vi "TEST FGV User Event Reference Manager.vi"(8 "error in (no error)":errorcluster) -> (0 "error out":errorcluster)   [LabVIEW 2009]
doc: "This is one of two stub VIs that will be completed in the exercise so that you can test the operation of the FGV User Event Reference Manager.\n\nAAL 9/09"
uses:
  Shared/QDMH Poly VIs/QDMH POLY Enqueue String.vi
panel:
  in  "Queue Name":string
  in  "Fire User Event":bool
  in  "User Event Ref to Act Upon":u16(ring)
  in  "Delete User Event":bool
  in  "Add User Event":bool
  out "Message Display":string
  in  "Cancel":bool
  in  "OK":bool
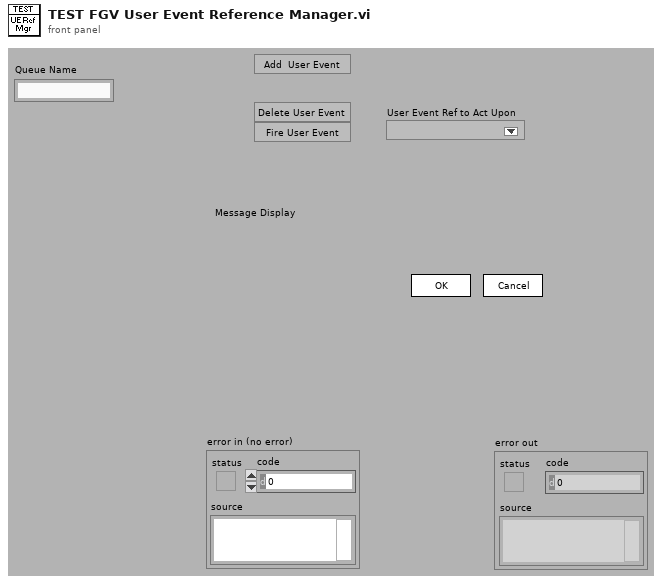
[diagram p1: front panel]
types:
  T1 = cluster{"Operator Name":string, "Current VI's Path":path, "# User Event  Refs":i32, "User Event #":i32, "User Event Names":string[], "User Event to Act Upon":i32}
  T2 = cluster{"User Event Name":string, "Variant":variant}
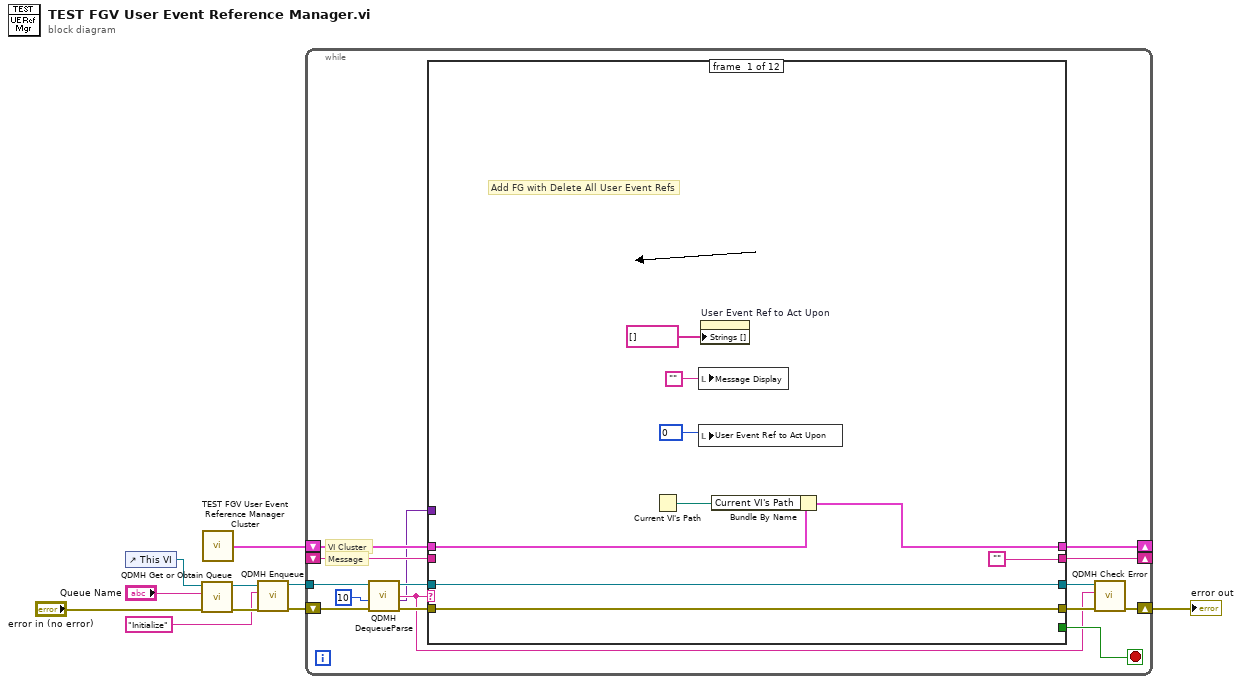
[diagram p0: block diagram]
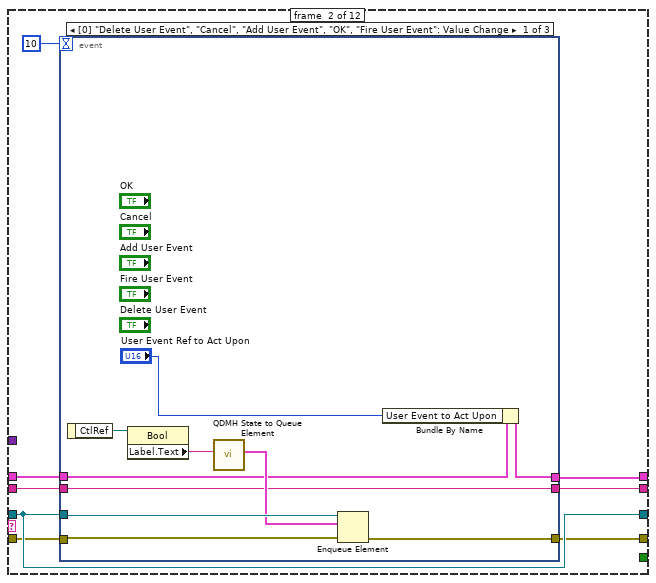
[diagram p2: hidden frame]
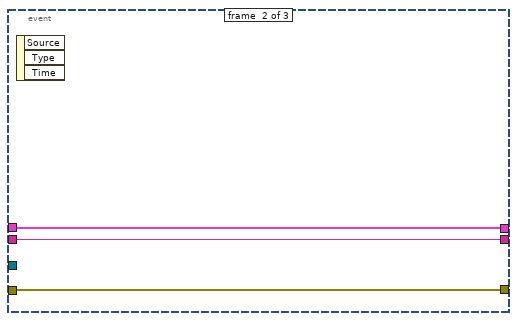
[diagram p3: hidden frame]
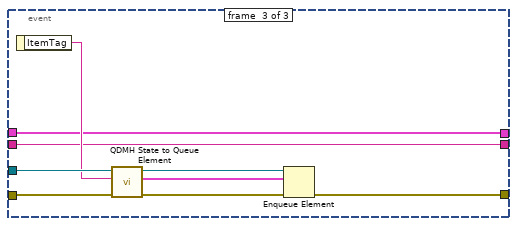
[diagram p4: hidden frame]
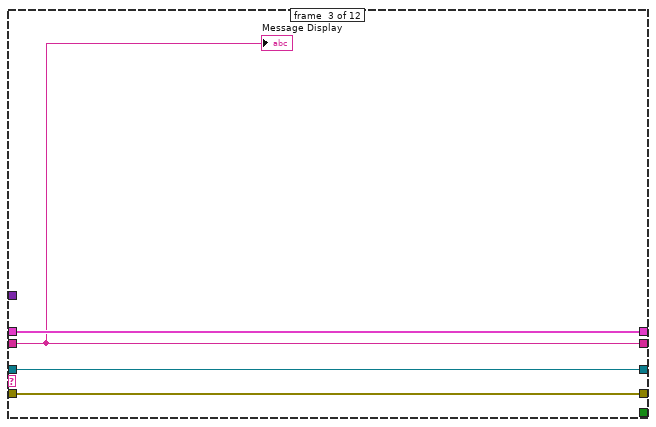
[diagram p5: hidden frame]
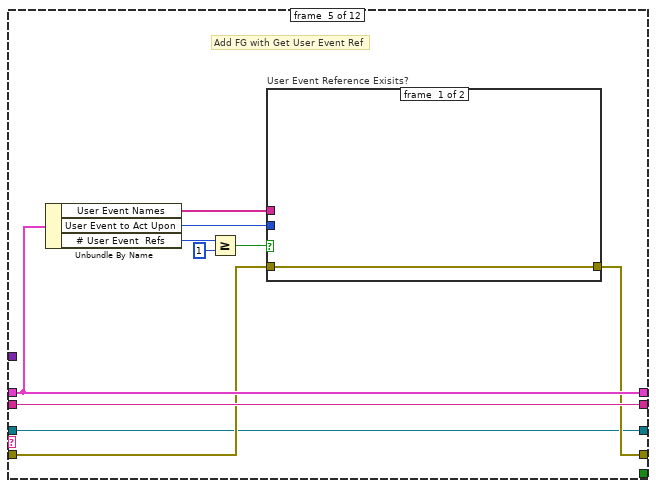
[diagram p7: hidden frame]
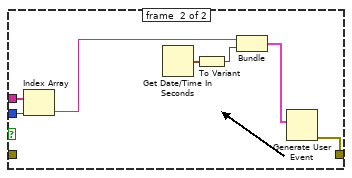
[diagram p8: hidden frame]
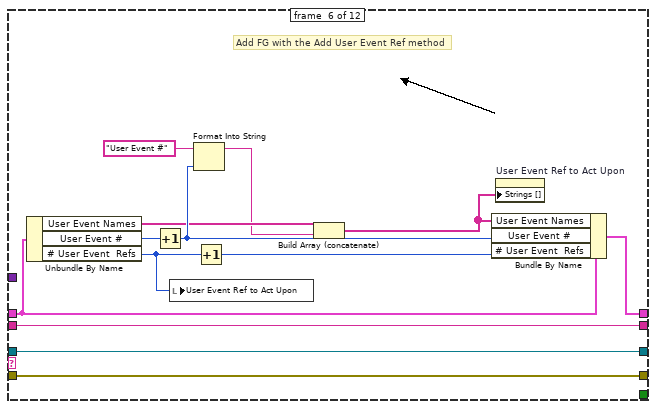
[diagram p9: hidden frame]
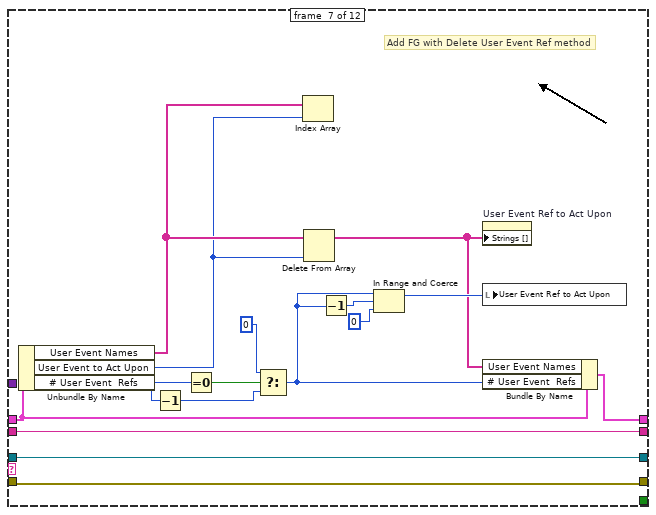
[diagram p10: hidden frame]
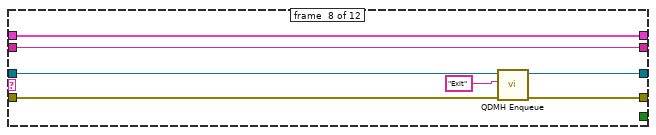
[diagram p11: hidden frame]
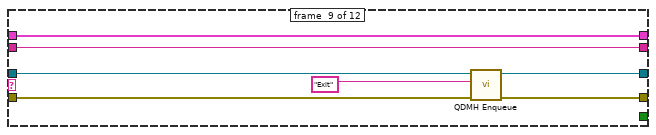
[diagram p12: hidden frame]
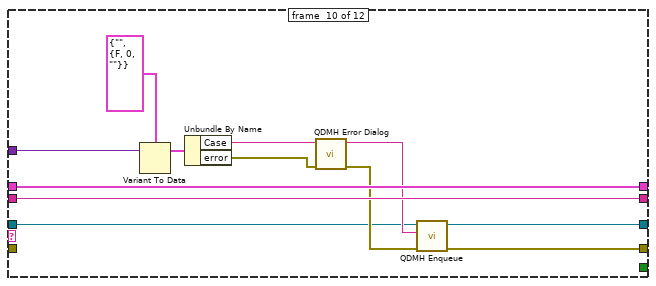
[diagram p13: hidden frame]
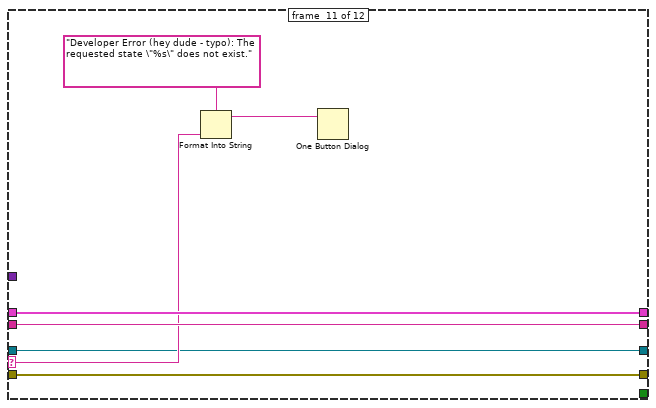
[diagram p14: hidden frame]
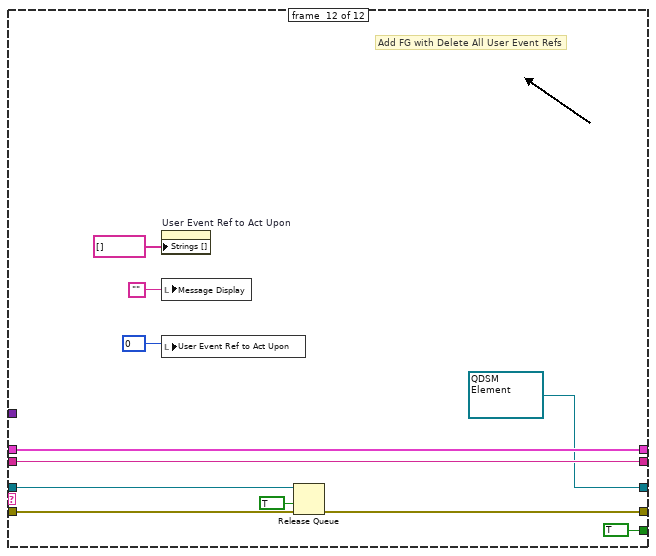
[diagram p15: hidden frame]
diagram:
  n1 = control-ref of="This VI"() -> (w2:refnum<vi>)
  n2 = call "QDMH Get or Obtain Queue.vi"("error in (no error)"="error in (no error)", "Queue Name"="Queue Name", "VI Refnum"=w2) -> ("error out"=w6:errorcluster, "queue out"=w9:refnum<queue>)  [unwired: 7 out]
  n3 = call "TEST FGV User Event Reference Manager Cluster.vi"() -> ("Cluster"=w8:T1)
  n4 = call-poly "QDMH Enqueue.vi"("error in (no error)"=w6, "State"="Initialize" ("element"), "queue"=w9) -> ("error out"=w7:errorcluster, "queue out"=w10:refnum<queue>)  [unwired: 7 out]
  n5 = while {
    tunnel: w10 -> [w21]
    shift-left: w8 -> [w22]
    shift-right: [w23] -> _
    shift-left: _ -> [w24]
    shift-right: [w15] -> _
    shift-right: [w13] -> w4
    shift-left: w7 -> [w17]
    stop <- w25 stop-if-true
    # "VI Cluster"
    # "Message"
    n6 = call "QDMH DequeueParse.vi"("error in (no error)"=w17, "Timeout"=10 ("ms timeout (-1)"), "queue"=w21) -> ("error out"=w18:errorcluster, "Variant Data"=w11:variant, "State"=w12:string, "queue out"=w19:refnum<queue>)  [unwired: 5 out]
    n7 = case shown="\"Initialize\"" w12 {
      selector: w12 -> [_ _ _ _ _ _ _ _ _ _ w147 _]
      tunnel: w19 -> [w26 w42 w63 w67 w71 w90 w102 w124 w131 w133 w144 w152]
      tunnel: [_ _ _ _ _ _ _ _ _ _ _ TRUE] -> w25
      tunnel: ["" w36 w65 w70 w80 w101 w117 w123 w130 w143 w150 w160] -> w15
      tunnel: w24 -> [_ w37 w65 w70 w80 w101 w117 w123 w130 w143 w150 w160]
      tunnel: [w32 w35 w66 w69 w79 w98 w115 w122 w129 w142 w149 w159] -> w23
      tunnel: w22 -> [w33 w38 w66 w69 w79 w99 w116 w122 w129 w142 w149 w159]
      tunnel: w18 -> [w34 w41 w64 w68 w76 w91 w104 w121 w128 _ w146 w157]
      tunnel: [w34 w40 w64 w68 w75 w91 w104 w120 w127 w134 w146 w156] -> w16
      tunnel: [w26 w42 w63 w67 w71 w90 w102 w118 w125 w135 w144 refnum<queue> refnum ("queue out")] -> w14
      tunnel: w11 -> [_ _ _ _ _ _ _ _ _ w132 _ _]
      frame #0 {
        w27 = u16 0 items=[""] ("Queue to Delete")
        # "Add FG with Delete All User Event Refs"
        n8 = Current VI's Path() -> (path=w31:path)
        n9 = local write "Message Display"("") -> ()
        n10 = local write "User Event Ref to Act Upon"(w27) -> ()
        n11 = property on="User Event Ref to Act Upon" class="Ring (strict)"("Strings []"=string[] []) -> ()  [unwired: 2 in, 2 out]
        n12 = Bundle By Name(cluster=w33, "Current VI's Path"=w31) -> (w32:T1)
      }
      frame #1 {
        n13 = event shown="[0] \"Delete User Event\", \"Cancel\", \"Add User Event\", \"OK\", \"Fire User Event\": Value Change" {
          selector: _ -> [_ _ _]
          dyn-events: _ -> [_ _ _]
          timeout: 10 -> [_ _ _]
          tunnel: w42 -> [w51 _ w62]
          tunnel: [w50 w55 w60] -> w40
          tunnel: w41 -> [w49 w55 w61]
          tunnel: w38 -> [w45 w54 w57]
          tunnel: w37 -> [w46 w53 w56]
          tunnel: [w44 w54 w57] -> w35
          tunnel: [w46 w53 w56] -> w36
          event #0 {
            n14 = event-data() -> ("CtlRef"=w52:refnum<vi>)  [unwired: 1 out]
            n15 = property class="Bool"(reference=w52) -> ("Label.Text"=w48:string)  [unwired: 1 in, 2 out]
            n16 = call "QDMH State to Queue Element.vi"("State"=w48) -> ("QDSM Element"=w47:cluster{"State":string, "Variant Data":variant})  [unwired: 10 out]
            n17 = Enqueue Element(queue=w51, element=w47, error in (no error)=w49) -> (error out=w50:errorcluster)  [unwired: 3 out]
            n18 = Bundle By Name(cluster=w45, "User Event to Act Upon"="User Event Ref to Act Upon") -> (w44:T1)
          }
          event #1 {
            n19 = event-data() -> ()  [unwired: 4 out]
          }
          event #2 {
            n20 = event-data() -> ("ItemTag"=w59:string)  [unwired: 1 out]
            n21 = call "QDMH State to Queue Element.vi"("State"=w59) -> ("QDSM Element"=w58:cluster{"State":string, "Variant Data":variant})  [unwired: 10 out]
            n22 = Enqueue Element(queue=w62, element=w58, error in (no error)=w61) -> (error out=w60:errorcluster)  [unwired: 3 out]
          }
        }
      }
      frame #2 {
        "Message Display" <- w65
      }
      frame #3 {
      }
      frame #4 {
        # "Add FG with Get User Event Ref"
        n23 = Unbundle By Name(w79) -> ("User Event Names"=w78:string[], "User Event to Act Upon"=w77:i32, "# User Event  Refs"=w74:i32)
        n24 = Greater Or Equal?(x=w74, y=1) -> (x >= y?=w72:bool)
        n25 = case "User Event Reference Exisits?" shown="True" w72 {
          tunnel: w78 -> [_ w88]
          tunnel: w77 -> [_ w84]
          tunnel: w76 -> [w81 _]
          tunnel: [w81 w83] -> w75
          frame #0 {
          }
          frame #1 {
            n26 = Index Array(array=w88, index=w84) -> (element=w82:string)
            n27 = Get Date/Time In Seconds() -> (seconds since 1Jan1904=w87:timestamp)
            n28 = To Variant(anything=w87) -> (Variant=w86:variant)
            n29 = Bundle("User Event Name"=w82, "Variant"=w86) -> (w85:T2)  [unwired: 1 out]
            n30 = Generate User Event(event data cluster=w85) -> (error out=w83:errorcluster)  [unwired: 2 in, 1 out]
          }
        }
      }
      frame #5 {
        # "Add FG with the Add User Event Ref method"
        n31 = Unbundle By Name(w99) -> ("User Event Names"=w94:string[], "User Event #"=w97:i32, "# User Event  Refs"=w92:i32)
        n32 = Increment(x=w97) -> (x+1=w96:i32)
        n33 = local write "User Event Ref to Act Upon"(w92) -> ()
        n34 = Format Into String(initial string="User Event #", w96) -> (resulting string=w89:string)  [unwired: 2 in, 1 out]
        n35 = Increment(x=w92) -> (x+1=w95:i32)
        n36 = Build Array (concatenate)(w94, w89) -> (w93:string[])
        n37 = Bundle By Name(cluster=w99, "User Event Names"=w93, "User Event #"=w96, "# User Event  Refs"=w95) -> (w98:T1)
        n38 = property on="User Event Ref to Act Upon" class="Ring (strict)"("Strings []"=w93) -> ()  [unwired: 2 in, 2 out]
      }
      frame #6 {
        # "Add FG with Delete User Event Ref method"
        n39 = Unbundle By Name(w116) -> ("User Event Names"=w106:string[], "User Event to Act Upon"=w105:i32, "# User Event  Refs"=w113:i32)
        n40 = Decrement(x=w113) -> (x-1=w111:i32)
        n41 = Equal To 0?(x=w113) -> (x = 0?=w114:bool)
        n42 = Select(t=0 ("# Queue Refs"), s=w114, f=w111) -> (s? t:f=w108:i32)
        n43 = Index Array(array=w106, index=w105) -> ()  [unwired: 1 out]
        n44 = Delete From Array(array=w106, index=w105) -> (array with subset deleted=w103:string[])  [unwired: 1 in, 1 out]
        n45 = Decrement(x=w108) -> (x-1=w110:i32)
        n46 = In Range and Coerce(upper limit=w108, x=w110, lower limit=0) -> (coerced(x)=w107:i32)  [unwired: 1 out]
        n47 = property on="User Event Ref to Act Upon" class="Ring (strict)"("Strings []"=w103) -> ()  [unwired: 2 in, 2 out]
        n48 = local write "User Event Ref to Act Upon"(w107) -> ()
        n49 = Bundle By Name(cluster=w116, "User Event Names"=w103, "# User Event  Refs"=w108) -> (w115:T1)
      }
      frame #7 {
        n50 = call-poly "QDMH Enqueue.vi"("error in (no error)"=w121, "State"="Exit" ("New State"), "queue"=w124) -> ("error out"=w120:errorcluster, "queue out"=w118:refnum<queue>)  [unwired: 7 out]
      }
      frame #8 {
        n51 = call-poly "QDMH Enqueue.vi"("error in (no error)"=w128, "State"="Exit" ("New State"), "queue"=w131) -> ("error out"=w127:errorcluster, "queue out"=w125:refnum<queue>)  [unwired: 7 out]
      }
      frame #9 {
        n52 = Variant To Data(Variant=w132, type=cluster{"Case":string, "error":errorcluster} {"Case"="", "error"={"status"=FALSE, "code"=0, "source"=""}} ("QDSM Element")) -> (data=w137:cluster{"Case":string, "error":errorcluster})  [unwired: 1 in, 1 out]
        n53 = Unbundle By Name(w137) -> ("Case"=w138:string, "error"=w139:errorcluster)
        n54 = call "QDMH Error Dialog.vi"("error"=w139, "Case Error Occured"=w138) -> ("error out (no error)"=w141:errorcluster, "Case to Execute"=w140:string)  [unwired: 8 out]
        n55 = call-poly "QDMH Enqueue.vi"("error in (no error)"=w141, "State"=w140, "queue"=w133) -> ("error out"=w134:errorcluster, "queue out"=w135:refnum<queue>)  [unwired: 7 out]
      }
      frame #10 {
        n56 = Format Into String(format string="Developer Error (hey dude - typo): The requested state \"%s\" does not exist." ("message"), w147) -> (resulting string=w145:string)  [unwired: 2 in, 1 out]
        n57 = One Button Dialog(message=w145) -> ()  [unwired: 2 out]
      }
      frame #11 {
        w153 = u16 0 items=[""] ("Queue to Delete")
        # "Add FG with Delete All User Event Refs"
        n58 = property on="User Event Ref to Act Upon" class="Ring (strict)"("Strings []"=string[] []) -> ()  [unwired: 2 in, 2 out]
        n59 = local write "Message Display"("") -> ()
        n60 = local write "User Event Ref to Act Upon"(w153) -> ()
        n61 = Release Queue(queue=w152, force destroy? (F)=TRUE, error in (no error)=w157) -> (error out=w156:errorcluster)  [unwired: 2 out]
      }
    }
    n62 = call "QDMH Check Error.vi"("error in (no error)"=w16, "Case"=w12, "queue"=w14) -> ("error out"=w13:errorcluster)  [unwired: 1 in, 7 out]
  }
  "error out" <- w4
